vi "AudioStreamer.Set Trainer.vi"(0 "destination":string, 7 "data":dbl[](array[numeric]), 11 "error in (no error)":errorcluster) -> (15 "error out":errorcluster)   [LabVIEW 2020]
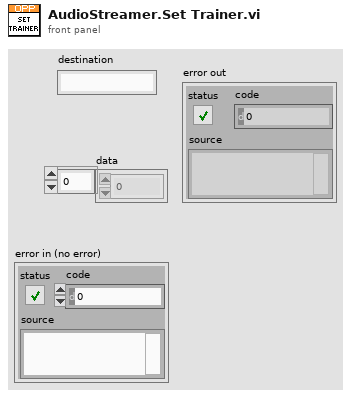
[diagram p1: front panel]
types:
  T1 = cluster{"destination":string, string, "data":dbl[]}
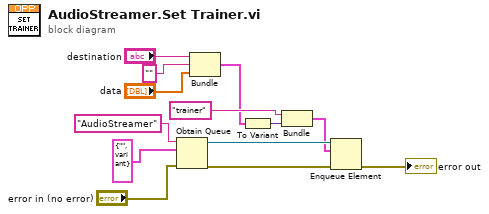
[diagram p0: block diagram]
diagram:
  n1 = Obtain Queue(name (unnamed)="AudioStreamer", element data type=cluster{string, variant} {"", variant}, error in (no error)="error in (no error)") -> (queue out=w10:refnum<queue>, error out=w11:errorcluster)  [unwired: 2 in, 1 out]
  n2 = Bundle("destination"="destination", "", "data"="data") -> (w4:T1)  [unwired: 1 in]
  n3 = To Variant(anything=w4) -> (Variant=w8:variant)
  n4 = Bundle("trainer", "Variant"=w8) -> (w6:cluster{string, "Variant":variant})  [unwired: 1 in]
  n5 = Enqueue Element(queue=w10, element=w6, error in (no error)=w11) -> (error out=→"error out":errorcluster)  [unwired: 1 in, 2 out]
